vi "Laboratoire 1.vi"() -> ()   [LabVIEW 2020]
panel:
  out "time left":i32
  out "données":dbl
  out "data":dynamicdata(graph) caption="données"
  in  "stop (F)":bool
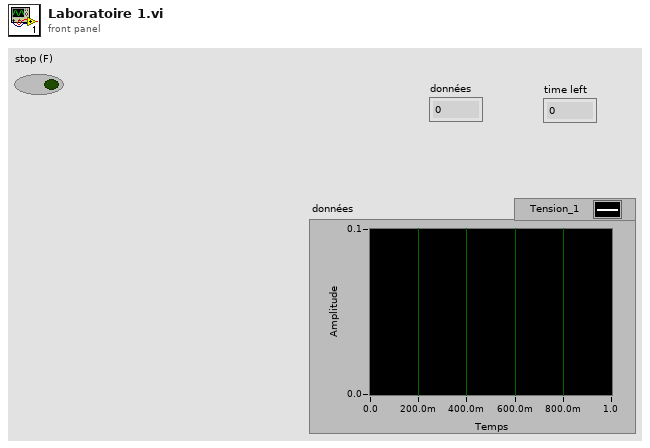
[diagram p1: front panel]
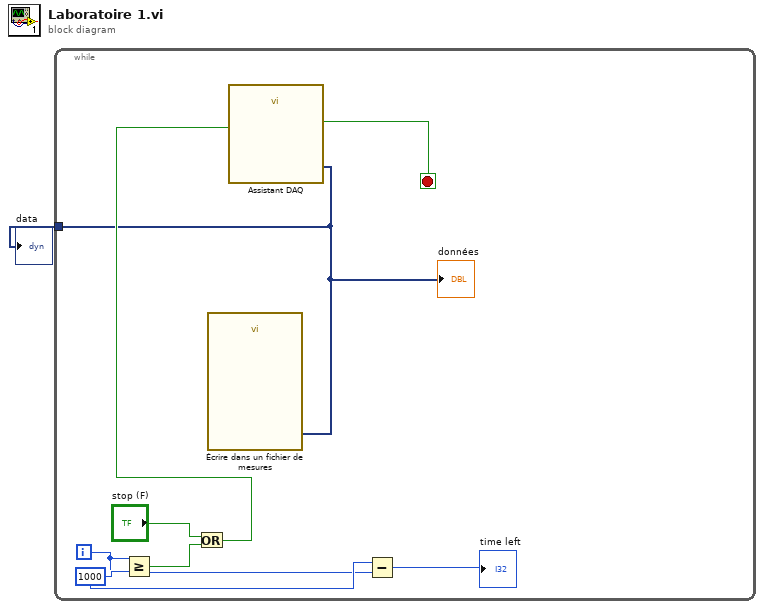
[diagram p0: block diagram]
diagram:
  n1 = while {
    tunnel: [w2] -> w1
    i -> [w4]
    stop <- w9 stop-if-true
    w5 = 1000
    n2 = Greater Or Equal?(x=w4, y=w5) -> (x >= y?=w7:bool)
    n3 = Or(x="stop (F)", y=w7) -> (x .or. y?=w6:bool)
    n4 = call "Assistant DAQ"("stop (F)"=w6) -> ("data"=w2:dynamicdata, "stopped"=w9:bool)  [unwired: 15 in, 2 out]
    "données" <- w2
    n5 = call "Écrire dans un fichier de mesures"("Signals"=w2) -> ()  [unwired: 16 in, 3 out]
    n6 = Subtract(x=w5, y=w4) -> (x-y=→"time left":i32)
  }
  "data" <- w1
